vi "test.vi"() -> ()   [LabVIEW 2019]
uses:
  Generated_client/RPC Messages/helloworld_HelloReply.ctl
  Generated_client/RPC Messages/helloworld_HelloRequest.ctl
  Generated_client/Generated_client.lvlib
panel:
  out "error out":errorcluster
  out "Response Data":T1
  in  "timeout (ms)":i32=-1
  in  "address":string
  in  "error in":errorcluster
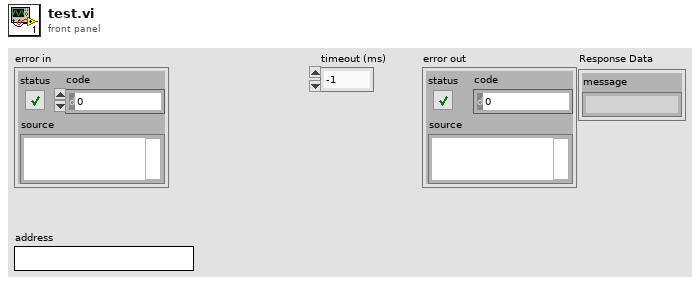
[diagram p1: front panel]
types:
  T1 = typedef "Generated_client.lvlib/helloworld_HelloReply.ctl" = cluster{"message":string}
  T2 = typedef "Generated_client.lvlib/helloworld_HelloRequest.ctl" = cluster{"name":string}
  T3 = typedef "grpc-lvsupport-release.lvlib/grpcId.ctl" = u64
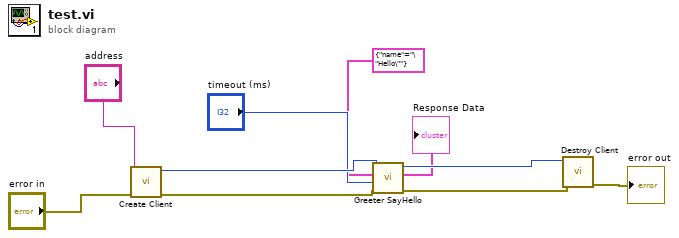
[diagram p0: block diagram]
diagram:
  n1 = call "Create Client.vi"("error in"="error in", "address"="address") -> ("error out"=w3:errorcluster, "gRPC ID Out"=w8:T3)  [unwired: 8 in]
  n2 = call "Greeter SayHello.vi"("error in"=w3, "timeout (ms)"="timeout (ms)", "Request Data"=T2 {"name"="\"Hello\""}, "gRPC ID"=w8) -> ("error out"=w2:errorcluster, "Response Data"=→"Response Data":T1, "gRPC ID out"=w7:T3)  [unwired: 5 in]
  n3 = call "Destroy Client.vi"("error in"=w2, "gRPC ID"=w7) -> ("error out"=→"error out":errorcluster)  [unwired: 9 in]
